vi "Server.vi"() -> ()   [LabVIEW 2023]
uses:
  <vilib>/Utility/file.llb/Read Delimited Spreadsheet (string).vi
  <vilib>/Utility/file.llb/Write Delimited Spreadsheet (string).vi
panel:
  in  "Tab Control":enum32{"CarWash", "Admin"}(tab)
  out "Vehicle Out of Position":bool
  out "Air Dry":bool
  out "Clean Water Rinse":bool
  out "Main High Pressure Wash":bool
  out "Soap Application":bool
  out "Under Body Wash":bool
  in  "Deluxe Wash":bool
  in  "Econony Wash":bool
  in  "Under body\nWash Position\nSwitch":bool
  in  "Main Wash\nPosition\nSwitch":bool
  in  "Air Dry\nPosition\nSwitch":bool
  in  "stop":bool
  out "Timer":i32
  in  "Users":string[][](array[string])
  in  "Read":bool
  in  "Save":bool
  in  "stop 2":bool
  out "Log":bool
  out "Count":bool
  # "Purchase Selection"
  # "Car Wash Indicators"
  # "Car Wash Simulation Switches"
  # "Username"
  # "Password"
  # "Role"
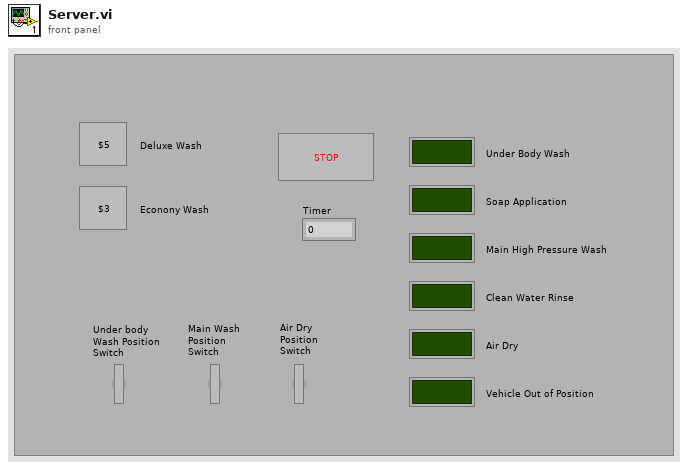
[diagram p1: front panel]
types:
  T1 = enum8{"Enabled", "Disabled", "Disabled and Grayed Out"}
  T2 = enum16{"Innit", "UBW", "SA", "MHPW", "CWR", "ADC"}
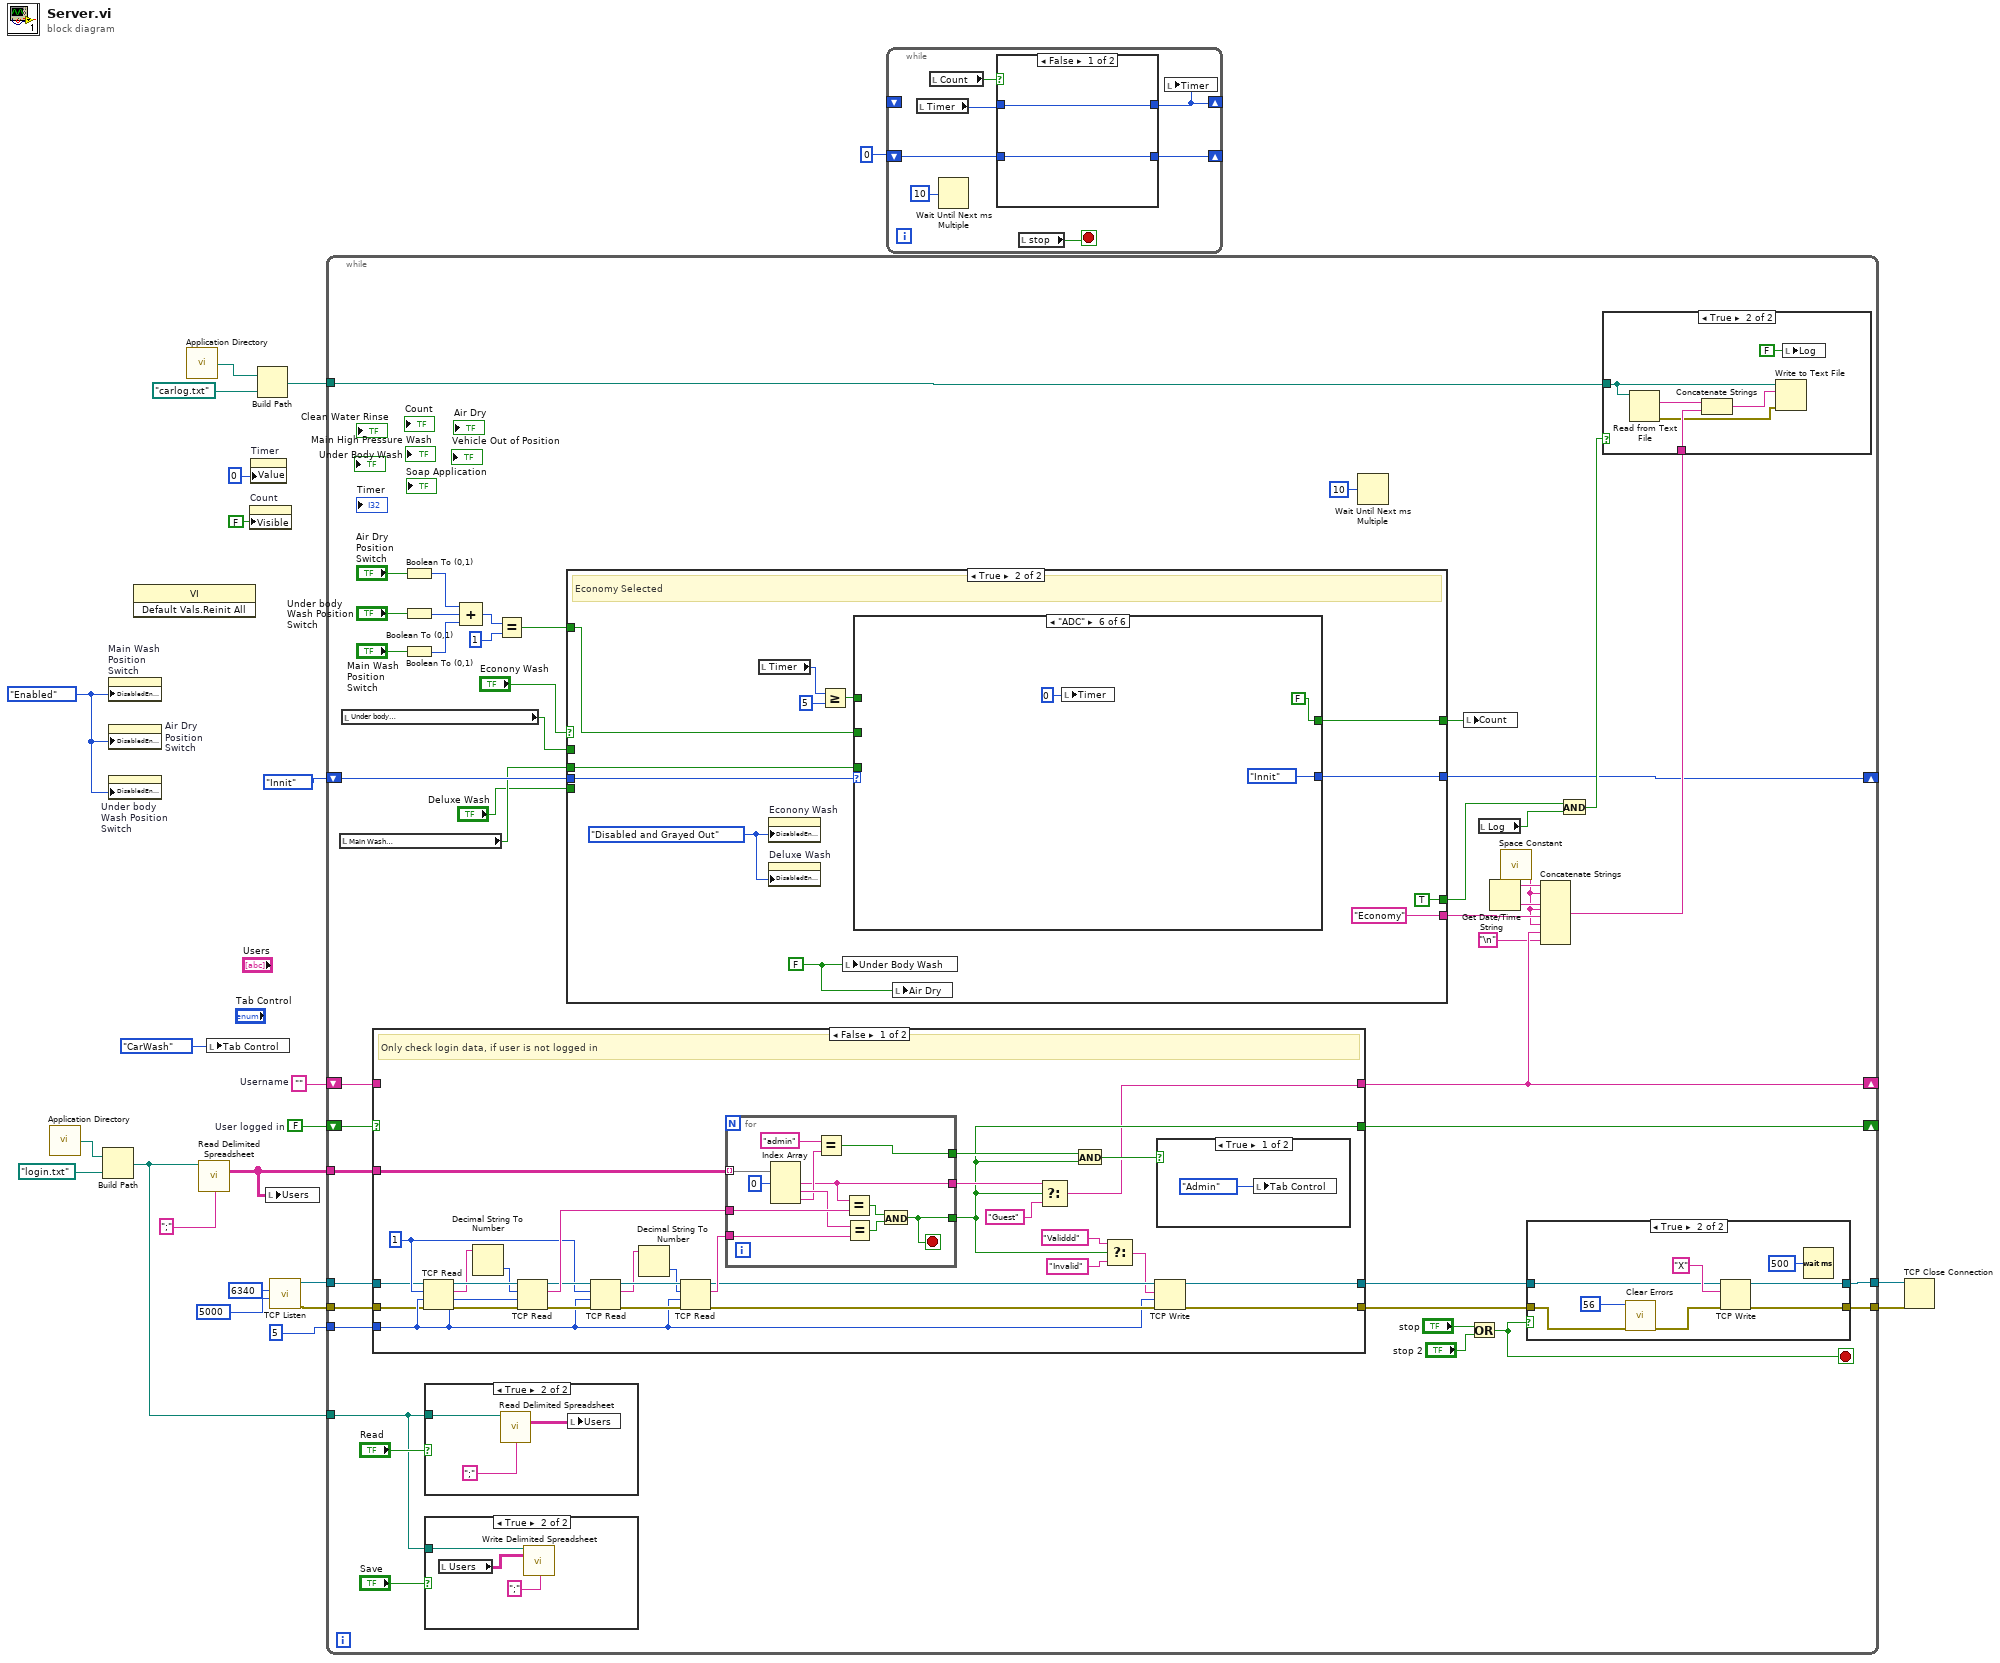
[diagram p0: block diagram]
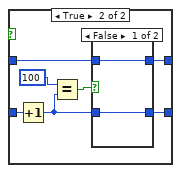
[diagram p2: hidden frame]
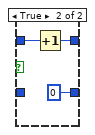
[diagram p3: hidden frame]
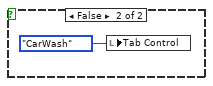
[diagram p6: hidden frame]
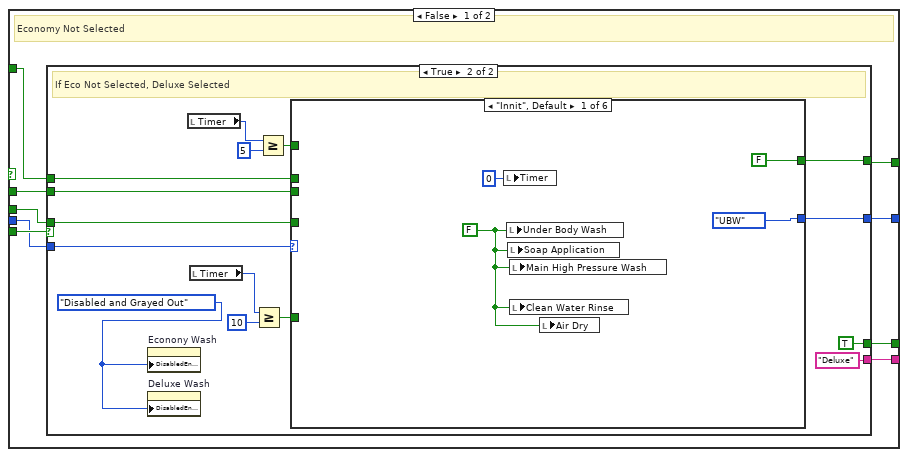
[diagram p10: hidden frame]
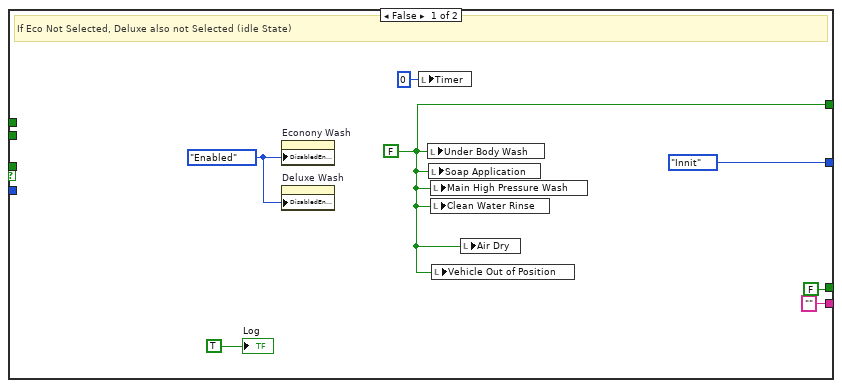
[diagram p11: hidden frame]
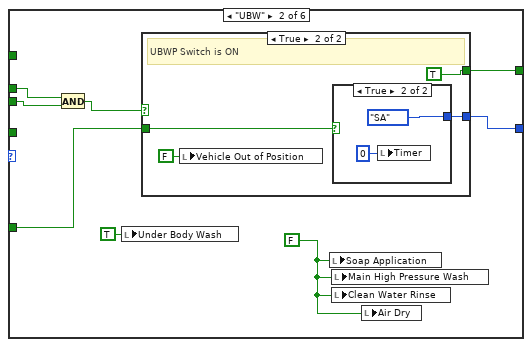
[diagram p12: hidden frame]
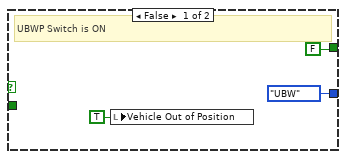
[diagram p13: hidden frame]
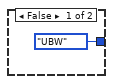
[diagram p14: hidden frame]
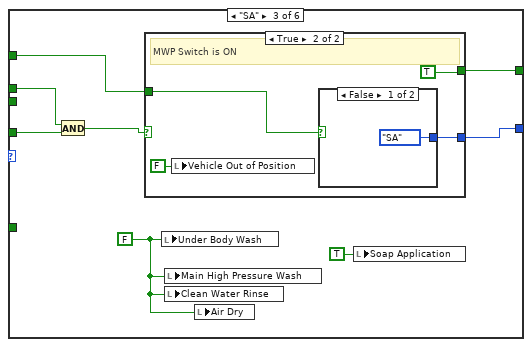
[diagram p15: hidden frame]
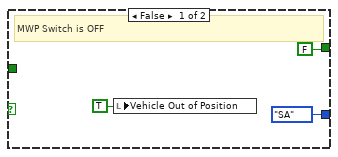
[diagram p16: hidden frame]
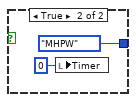
[diagram p17: hidden frame]
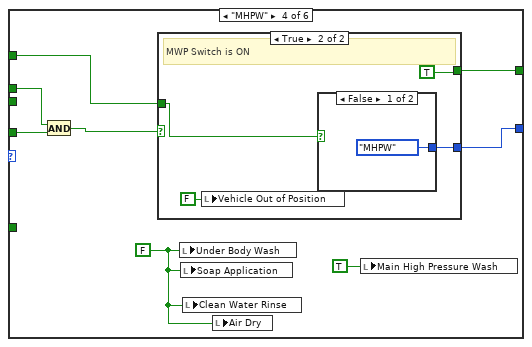
[diagram p18: hidden frame]
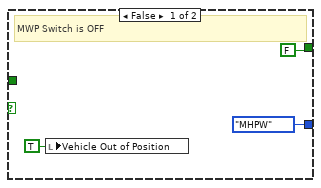
[diagram p19: hidden frame]
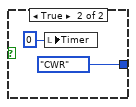
[diagram p20: hidden frame]
diagram:
  w1 = T1."Enabled" ("Disabled")
  w3 = ""  # Username
  w8 = FALSE  # User logged in
  n1 = call <vilib>:"Application Directory.vi"() -> ("Application Directory"=w9:path)
  n2 = Build Path(base path=w9, name or relative path=path "login.txt") -> (appended path=w5:path)
  n3 = property on="Main Wash\nPosition\nSwitch" class="Bool (strict)"("DisabledEnum"=w1) -> ()  [unwired: 2 in, 2 out]
  n4 = property on="Air Dry\nPosition\nSwitch" class="Bool (strict)"("DisabledEnum"=w1) -> ()  [unwired: 2 in, 2 out]
  n5 = property on="Under body\nWash Position\nSwitch" class="Bool (strict)"("DisabledEnum"=w1) -> ()  [unwired: 2 in, 2 out]
  n6 = invoke class="VI" method="Default Vals.Reinit All"() -> ()  [unwired: 3 in, 3 out]
  n7 = call <vilib>:"Application Directory.vi"() -> ("Application Directory"=w13:path)
  n8 = call-poly <vilib>:"Read Delimited Spreadsheet.vi"("file path (dialog if empty)"=w5, "delimiter (\\t)"=";" ("delimiter (\\t)")) -> ("all rows"=w6:string[][])  [unwired: 8 in, 5 out]
  n9 = local write "Tab Control"(enum32{"CarWash", "Admin"}."CarWash" ("Tab Control")) -> ()
  n10 = property on="Count" class="Bool (strict)"("Visible"=FALSE ("Count")) -> ()  [unwired: 2 in, 2 out]
  n11 = property on="Timer" class="DigNum (strict)"("Value"=0 ("Timer")) -> ()  [unwired: 2 in, 2 out]
  n12 = Build Path(base path=w13, name or relative path=path "carlog.txt") -> (appended path=w2:path)
  n13 = local write "Users"(w6) -> ()
  n14 = call <vilib>:"TCP Listen.vi"("timeout ms (wait forever: -1)"=5000 ("timeout ms (60000)"), "port"=u16 6340) -> ("error out"=w16:errorcluster, "connection ID"=w19:refnum<k5>)  [unwired: 5 in, 3 out]
  n15 = while {
    shift-right: [w53] -> _
    shift-left: T2."Innit" -> [w68]
    tunnel: w2 -> [w56]
    tunnel: w19 -> [w51]
    tunnel: [w47] -> w18
    tunnel: [w46] -> w17
    tunnel: w16 -> [w50]
    tunnel: 5 ("timeout ms (60000)") -> [w52]
    shift-right: [w44] -> _
    shift-left: w8 -> [w45]
    tunnel: w6 -> [w43]
    tunnel: w5 -> [w37]
    shift-right: [w34] -> _
    shift-left: w3 -> [w36]
    stop <- w40 stop-if-true
    n16 = local read "Main Wash\nPosition\nSwitch"() -> (w67:bool)
    n17 = local read "Under body\nWash Position\nSwitch"() -> (w66:bool)
    n18 = case shown="False" w45 {
      selector: w45 -> [_ w120]
      tunnel: w52 -> [w86 _]
      tunnel: w51 -> [w85 w122]
      tunnel: w50 -> [w84 w121]
      tunnel: [w83 w121] -> w49
      tunnel: [w82 w122] -> w48
      tunnel: [w77 w120] -> w44
      tunnel: w43 -> [w81 _]
      tunnel: w36 -> [_ w119]
      tunnel: [w75 w119] -> w34
      frame False {
        w87 = 1
        # "Only check login data, if user is not logged in"
        n19 = TCP Read(connection ID=w85, bytes to read=w87, error in (no error)=w84, 9:w86) -> (connection ID out=w97:refnum<k5>, data out=w95:string, error out=w96:errorcluster)  [unwired: 1 in]
        n20 = Decimal String To Number(string=w95) -> (number=w94:i32)  [unwired: 2 in, 1 out]
        n21 = TCP Read(connection ID=w97, bytes to read=w94, error in (no error)=w96, 9:w86) -> (connection ID out=w90:refnum<k5>, data out=w104:string, error out=w91:errorcluster)  [unwired: 1 in]
        n22 = TCP Read(connection ID=w90, bytes to read=w87, error in (no error)=w91, 9:w86) -> (connection ID out=w93:refnum<k5>, data out=w89:string, error out=w92:errorcluster)  [unwired: 1 in]
        n23 = Decimal String To Number(string=w89) -> (number=w88:i32)  [unwired: 2 in, 1 out]
        n24 = TCP Read(connection ID=w93, bytes to read=w88, error in (no error)=w92, 9:w86) -> (connection ID out=w100:refnum<k5>, data out=w103:string, error out=w99:errorcluster)  [unwired: 1 in]
        n25 = for {
          tunnel: w104 -> [w117]
          tunnel: w103 -> [w116]
          tunnel: w81 -> [w118] mode=indexing
          tunnel: [w111] -> w77
          tunnel: [w108] -> w80
          tunnel: [w107] -> w78
          stop <- w111 stop-if-true
          n26 = Index Array(array=w118, index #1=0 ("index")) -> (element #1=w107:string, element #2=w114:string, element #3=w110:string)  [unwired: 2 in]
          n27 = Equal?(x="admin", y=w110) -> (x = y?=w108:bool)
          n28 = Equal?(x=w107, y=w117) -> (x = y?=w112:bool)
          n29 = Equal?(x=w114, y=w116) -> (x = y?=w113:bool)
          n30 = And(x=w112, y=w113) -> (x .and. y?=w111:bool)
        }
        n31 = Select(t=w78, s=w77, f="Guest") -> (s? t:f=w75:string)
        n32 = And(x=w80, y=w77) -> (x .and. y?=w79:bool)
        n33 = Select(t="Validdd", s=w77, f="Invalid") -> (s? t:f=w98:string)
        n34 = TCP Write(connection ID=w100, data in=w98, error in (no error)=w99, 9:w86) -> (connection ID out=w82:refnum<k5>, error out=w83:errorcluster)  [unwired: 1 out]
        n35 = case shown="True" w79 {
          frame True {
            n36 = local write "Tab Control"(enum32{"CarWash", "Admin"}."Admin" ("Tab Control")) -> ()
          }
          frame False {
            n37 = local write "Tab Control"(enum32{"CarWash", "Admin"}."CarWash" ("Tab Control")) -> ()
          }
        }
      }
      frame True {
        # "When logged in, there is nothig to do here"
      }
    }
    n38 = Boolean To (0,1)(Boolean="Air Dry\nPosition\nSwitch") -> (0, 1=w29:i16)
    n39 = Boolean To (0,1)(Boolean="Under body\nWash Position\nSwitch") -> (0, 1=w28:i16)
    n40 = Boolean To (0,1)(Boolean="Main Wash\nPosition\nSwitch") -> (0, 1=w27:i16)
    n41 = case shown="True" "Read" {
      tunnel: w37 -> [_ w72]
      frame False {
      }
      frame True {
        n42 = call-poly <vilib>:"Read Delimited Spreadsheet.vi"("file path (dialog if empty)"=w72, "delimiter (\\t)"=";" ("delimiter (\\t)")) -> ("all rows"=w74:string[][])  [unwired: 8 in, 5 out]
        n43 = local write "Users"(w74) -> ()
      }
    }
    n44 = case shown="True" "Save" {
      tunnel: w37 -> [_ w70]
      frame False {
      }
      frame True {
        n45 = local read "Users"() -> (w69:string[][])
        n46 = call-poly <vilib>:"Write Delimited Spreadsheet.vi"("file path (dialog if empty)"=w70, "2D data"=w69, "delimiter (\\t)"=";" ("delimiter (\\t)")) -> ()  [unwired: 11 in, 2 out]
      }
    }
    n47 = Compound Arithmetic op=ADD(w29, w28, w27) -> (w26:i16)
    n48 = Equal?(x=w26, y=i16 1) -> (x = y?=w24:bool)
    n49 = case shown="True" "Econony Wash" {
      tunnel: w68 -> [w146 w275]
      tunnel: "Deluxe Wash" -> [w147 _]
      tunnel: [w145 w274] -> w53
      tunnel: w67 -> [w143 w272]
      tunnel: w66 -> [w144 _]
      tunnel: [w142 w271] -> w63
      tunnel: [w141 "Economy"] -> w55
      tunnel: [w140 TRUE] -> w54
      tunnel: w24 -> [w139 w264]
      frame False {
        # "Economy Not Selected"
        n50 = case shown="True" w147 {
          tunnel: w146 -> [_ w169]
          tunnel: [T2."Innit" w168] -> w145
          tunnel: w144 -> [_ w167]
          tunnel: w143 -> [_ w166]
          tunnel: [w152 w161] -> w142
          tunnel: ["" "Deluxe"] -> w141
          tunnel: [FALSE TRUE] -> w140
          tunnel: w139 -> [_ w155]
          frame False {
            w148 = T1."Enabled" ("Disabled")
            w152 = FALSE ("Soap Application")
            # "If Eco Not Selected, Deluxe also not Selected (idle State)"
            n51 = property on="Econony Wash" class="Bool (strict)"("DisabledEnum"=w148) -> ()  [unwired: 2 in, 2 out]
            n52 = property on="Deluxe Wash" class="Bool (strict)"("DisabledEnum"=w148) -> ()  [unwired: 2 in, 2 out]
            n53 = local write "Timer"(0 ("Timer")) -> ()
            n54 = local write "Under Body Wash"(w152) -> ()
            n55 = local write "Soap Application"(w152) -> ()
            n56 = local write "Main High Pressure Wash"(w152) -> ()
            n57 = local write "Clean Water Rinse"(w152) -> ()
            n58 = local write "Vehicle Out of Position"(w152) -> ()
            n59 = local write "Air Dry"(w152) -> ()
            "Log" <- TRUE
          }
          frame True {
            w156 = T1."Disabled and Grayed Out" ("Disabled")
            # "If Eco Not Selected, Deluxe Selected"
            n60 = property on="Econony Wash" class="Bool (strict)"("DisabledEnum"=w156) -> ()  [unwired: 2 in, 2 out]
            n61 = property on="Deluxe Wash" class="Bool (strict)"("DisabledEnum"=w156) -> ()  [unwired: 2 in, 2 out]
            n62 = local read "Timer"() -> (w163:i32)
            n63 = local read "Timer"() -> (w162:i32)
            n64 = Greater Or Equal?(x=w162, y=10) -> (x >= y?=w160:bool)
            n65 = Greater Or Equal?(x=w163, y=5) -> (x >= y?=w159:bool)
            n66 = case shown="\"Innit\", Default" w169 {
              tunnel: [T2."UBW" w181 w199 w217 w234 w253] -> w168
              tunnel: w167 -> [_ w176 _ _ _ _]
              tunnel: w166 -> [_ _ w194 w212 w230 _]
              tunnel: [FALSE w178 w196 w214 w232 w249] -> w161
              tunnel: w160 -> [_ w177 _ _ _ w250]
              tunnel: w159 -> [_ _ w195 w213 w231 _]
              tunnel: w155 -> [_ w175 w192 w210 w228 w246]
              frame "Innit", Default {
                w172 = FALSE ("Soap Application")
                n67 = local write "Timer"(0 ("Timer")) -> ()
                n68 = local write "Under Body Wash"(w172) -> ()
                n69 = local write "Soap Application"(w172) -> ()
                n70 = local write "Main High Pressure Wash"(w172) -> ()
                n71 = local write "Clean Water Rinse"(w172) -> ()
                n72 = local write "Air Dry"(w172) -> ()
              }
              frame "UBW" {
                w179 = FALSE ("Soap Application")
                n73 = And(x=w175, y=w176) -> (x .and. y?=w174:bool)
                n74 = local write "Under Body Wash"(TRUE ("Soap Application")) -> ()
                n75 = case shown="True" w174 {
                  tunnel: [T2."UBW" w188] -> w181
                  tunnel: [FALSE TRUE] -> w178
                  tunnel: w177 -> [_ w185]
                  frame False {
                    # "UBWP Switch is ON"
                    n76 = local write "Vehicle Out of Position"(TRUE ("Vehicle Out of Position")) -> ()
                  }
                  frame True {
                    # "UBWP Switch is ON"
                    n77 = local write "Vehicle Out of Position"(FALSE ("Vehicle Out of Position")) -> ()
                    n78 = case shown="True" w185 {
                      tunnel: [T2."UBW" T2."SA"] -> w188
                      frame False {
                      }
                      frame True {
                        n79 = local write "Timer"(0 ("Timer")) -> ()
                      }
                    }
                  }
                }
                n80 = local write "Soap Application"(w179) -> ()
                n81 = local write "Main High Pressure Wash"(w179) -> ()
                n82 = local write "Clean Water Rinse"(w179) -> ()
                n83 = local write "Air Dry"(w179) -> ()
              }
              frame "SA" {
                w198 = FALSE ("Soap Application")
                n84 = And(x=w192, y=w194) -> (x .and. y?=w193:bool)
                n85 = case shown="True" w193 {
                  tunnel: [T2."SA" w206] -> w199
                  tunnel: [FALSE TRUE] -> w196
                  tunnel: w195 -> [_ w203]
                  frame False {
                    # "MWP Switch is OFF"
                    n86 = local write "Vehicle Out of Position"(TRUE ("Vehicle Out of Position")) -> ()
                  }
                  frame True {
                    # "MWP Switch is ON"
                    n87 = local write "Vehicle Out of Position"(FALSE ("Vehicle Out of Position")) -> ()
                    n88 = case shown="False" w203 {
                      tunnel: [T2."SA" T2."MHPW"] -> w206
                      frame False {
                      }
                      frame True {
                        n89 = local write "Timer"(0 ("Timer")) -> ()
                      }
                    }
                  }
                }
                n90 = local write "Under Body Wash"(w198) -> ()
                n91 = local write "Main High Pressure Wash"(w198) -> ()
                n92 = local write "Clean Water Rinse"(w198) -> ()
                n93 = local write "Air Dry"(w198) -> ()
                n94 = local write "Soap Application"(TRUE ("Soap Application")) -> ()
              }
              frame "MHPW" {
                w216 = FALSE ("Soap Application")
                n95 = And(x=w210, y=w212) -> (x .and. y?=w211:bool)
                n96 = case shown="True" w211 {
                  tunnel: [T2."MHPW" w224] -> w217
                  tunnel: [FALSE TRUE] -> w214
                  tunnel: w213 -> [_ w221]
                  frame False {
                    # "MWP Switch is OFF"
                    n97 = local write "Vehicle Out of Position"(TRUE ("Vehicle Out of Position")) -> ()
                  }
                  frame True {
                    # "MWP Switch is ON"
                    n98 = local write "Vehicle Out of Position"(FALSE ("Vehicle Out of Position")) -> ()
                    n99 = case shown="False" w221 {
                      tunnel: [T2."MHPW" T2."CWR"] -> w224
                      frame False {
                      }
                      frame True {
                        n100 = local write "Timer"(0) -> ()
                      }
                    }
                  }
                }
                n101 = local write "Under Body Wash"(w216) -> ()
                n102 = local write "Soap Application"(w216) -> ()
                n103 = local write "Clean Water Rinse"(w216) -> ()
                n104 = local write "Air Dry"(w216) -> ()
                n105 = local write "Main High Pressure Wash"(TRUE ("Soap Application")) -> ()
              }
              frame "CWR" {
                w233 = FALSE ("Soap Application")
                n106 = And(x=w228, y=w230) -> (x .and. y?=w229:bool)
                n107 = local write "Clean Water Rinse"(TRUE ("Soap Application")) -> ()
                n108 = local write "Under Body Wash"(w233) -> ()
                n109 = local write "Soap Application"(w233) -> ()
                n110 = local write "Main High Pressure Wash"(w233) -> ()
                n111 = local write "Air Dry"(w233) -> ()
                n112 = case shown="True" w229 {
                  tunnel: [T2."CWR" w242] -> w234
                  tunnel: [FALSE TRUE] -> w232
                  tunnel: w231 -> [_ w239]
                  frame False {
                    # "MWP Switch is OFF"
                    n113 = local write "Vehicle Out of Position"(TRUE ("Vehicle Out of Position")) -> ()
                  }
                  frame True {
                    # "MWP Switch is ON"
                    n114 = local write "Vehicle Out of Position"(FALSE ("Vehicle Out of Position")) -> ()
                    n115 = case shown="True" w239 {
                      tunnel: [T2."CWR" T2."ADC"] -> w242
                      frame False {
                      }
                      frame True {
                        n116 = local write "Timer"(0 ("Timer")) -> ()
                      }
                    }
                  }
                }
              }
              frame "ADC" {
                w252 = FALSE ("Soap Application")
                n117 = local read "Air Dry\nPosition\nSwitch"() -> (w248:bool)
                n118 = local write "Under Body Wash"(w252) -> ()
                n119 = local write "Soap Application"(w252) -> ()
                n120 = local write "Main High Pressure Wash"(w252) -> ()
                n121 = local write "Clean Water Rinse"(w252) -> ()
                n122 = local write "Air Dry"(TRUE ("Soap Application")) -> ()
                n123 = And(x=w246, y=w248) -> (x .and. y?=w247:bool)
                n124 = case shown="True" w247 {
                  tunnel: [T2."ADC" w260] -> w253
                  tunnel: w250 -> [_ w258]
                  tunnel: [FALSE TRUE] -> w249
                  frame False {
                    n125 = local write "Vehicle Out of Position"(TRUE ("Vehicle Out of Position")) -> ()
                  }
                  frame True {
                    n126 = local write "Vehicle Out of Position"(FALSE ("Vehicle Out of Position")) -> ()
                    n127 = case shown="True" w258 {
                      tunnel: [T2."ADC" T2."Innit"] -> w260
                      frame False {
                      }
                      frame True {
                        n128 = invoke class="VI" method="Default Vals.Reinit All"() -> ()  [unwired: 3 in, 3 out]
                        n129 = local write "Timer"(0 ("Timer")) -> ()
                      }
                    }
                  }
                }
              }
            }
          }
        }
      }
      frame True {
        w265 = T1."Disabled and Grayed Out" ("Disabled")
        w273 = FALSE ("Soap Application")
        # "Economy Selected"
        n130 = local read "Timer"() -> (w270:i32)
        n131 = property on="Econony Wash" class="Bool (strict)"("DisabledEnum"=w265) -> ()  [unwired: 2 in, 2 out]
        n132 = property on="Deluxe Wash" class="Bool (strict)"("DisabledEnum"=w265) -> ()  [unwired: 2 in, 2 out]
        n133 = Greater Or Equal?(x=w270, y=5) -> (x >= y?=w268:bool)
        n134 = local write "Under Body Wash"(w273) -> ()
        n135 = case shown="\"ADC\"" w275 {
          tunnel: [T2."SA" T2."Innit" w290 w308 w326 T2."Innit"] -> w274
          tunnel: w272 -> [_ _ w285 w303 w321 _]
          tunnel: [FALSE ("Count") FALSE ("Count") w287 w305 w322 FALSE ("Count")] -> w271
          tunnel: w268 -> [_ _ w286 w304 w323 _]
          tunnel: w264 -> [_ _ w284 w302 w319 _]
          frame "Innit", Default {
            w278 = FALSE ("Soap Application")
            n136 = local write "Main High Pressure Wash"(w278) -> ()
            n137 = local write "Clean Water Rinse"(w278) -> ()
            n138 = local write "Soap Application"(w278) -> ()
            n139 = local write "Timer"(0 ("Timer")) -> ()
          }
          frame "UBW" {
            n140 = local write "Timer"(0 ("Timer")) -> ()
          }
          frame "SA" {
            w288 = FALSE ("Soap Application")
            n141 = And(x=w284, y=w285) -> (x .and. y?=w283:bool)
            n142 = local write "Soap Application"(TRUE ("Soap Application")) -> ()
            n143 = local write "Main High Pressure Wash"(w288) -> ()
            n144 = case shown="True" w283 {
              tunnel: [T2."SA" w297] -> w290
              tunnel: [FALSE ("Count") TRUE ("Count")] -> w287
              tunnel: w286 -> [_ w294]
              frame False {
                # "MWP Switch is OFF"
                n145 = local write "Vehicle Out of Position"(TRUE ("Vehicle Out of Position")) -> ()
              }
              frame True {
                # "MWP Switch is ON"
                n146 = local write "Vehicle Out of Position"(FALSE ("Vehicle Out of Position")) -> ()
                n147 = case shown="False" w294 {
                  tunnel: [T2."SA" T2."MHPW"] -> w297
                  frame False {
                  }
                  frame True {
                    n148 = local write "Timer"(0 ("Timer")) -> ()
                  }
                }
              }
            }
            n149 = local write "Clean Water Rinse"(w288) -> ()
          }
          frame "MHPW" {
            w307 = FALSE ("Soap Application")
            n150 = local write "Main High Pressure Wash"(TRUE ("Soap Application")) -> ()
            n151 = And(x=w302, y=w303) -> (x .and. y?=w301:bool)
            n152 = local write "Clean Water Rinse"(w307) -> ()
            n153 = local write "Soap Application"(w307) -> ()
            n154 = case shown="False" w301 {
              tunnel: [T2."MHPW" w315] -> w308
              tunnel: [FALSE TRUE] -> w305
              tunnel: w304 -> [_ w312]
              frame False {
                # "MWP Switch is OFF"
                n155 = local write "Vehicle Out of Position"(TRUE ("Vehicle Out of Position")) -> ()
              }
              frame True {
                # "MWP Switch is ON"
                n156 = local write "Vehicle Out of Position"(FALSE ("Vehicle Out of Position")) -> ()
                n157 = case shown="True" w312 {
                  tunnel: [T2."MHPW" T2."CWR"] -> w315
                  frame False {
                  }
                  frame True {
                    n158 = local write "Timer"(0 ("Timer")) -> ()
                  }
                }
              }
            }
          }
          frame "CWR" {
            w324 = FALSE ("Soap Application")
            n159 = local write "Clean Water Rinse"(TRUE ("Soap Application")) -> ()
            n160 = And(x=w319, y=w321) -> (x .and. y?=w320:bool)
            n161 = local write "Main High Pressure Wash"(w324) -> ()
            n162 = local write "Soap Application"(w324) -> ()
            n163 = case shown="True" w320 {
              tunnel: [T2."CWR" w333] -> w326
              tunnel: w323 -> [_ w331]
              tunnel: [FALSE TRUE] -> w322
              frame False {
                # "MWP Switch is OFF"
                n164 = local write "Vehicle Out of Position"(TRUE ("Vehicle Out of Position")) -> ()
              }
              frame True {
                # "MWP Switch is ON"
                n165 = local write "Vehicle Out of Position"(FALSE ("Vehicle Out of Position")) -> ()
                n166 = case shown="True" w331 {
                  tunnel: [T2."CWR" T2."Innit"] -> w333
                  frame False {
                  }
                  frame True {
                    n167 = invoke class="VI" method="Default Vals.Reinit All"() -> ()  [unwired: 3 in, 3 out]
                    n168 = local write "Timer"(0 ("Timer")) -> ()
                  }
                }
              }
            }
          }
          frame "ADC" {
            n169 = local write "Timer"(0 ("Timer")) -> ()
          }
        }
        n170 = local write "Air Dry"(w273) -> ()
      }
    }
    n171 = Wait Until Next ms Multiple(millisecond multiple=u32 10) -> ()  [unwired: 1 out]
    n172 = local write "Count"(w63) -> ()
    n173 = Or(x="stop", y="stop 2") -> (x .or. y?=w40:bool)
    n174 = local read "Log"() -> (w60:bool)
    n175 = Get Date/Time String() -> (date string=w59:string, time string=w58:string)  [unwired: 3 in]
    n176 = call <vilib>:"Space Constant.vi"() -> ("String"=w35:string)
    n177 = case shown="True" w40 {
      tunnel: w49 -> [w123 w132]
      tunnel: w48 -> [w124 w126]
      tunnel: [w124 w131] -> w47
      tunnel: [w123 w130] -> w46
      frame False {
      }
      frame True {
        n178 = call <vilib>:"Clear Errors.vi"("error in (no error)"=w132, "specific error code to clear (0: all)"=56) -> ("error out"=w127:errorcluster)  [unwired: 4 in, 1 out]
        n179 = TCP Write(connection ID=w126, data in="X", error in (no error)=w127) -> (connection ID out=w131:refnum<k5>, error out=w130:errorcluster)  [unwired: 1 in, 1 out]
        n180 = Wait (ms)(milliseconds to wait=u32 500) -> ()  [unwired: 1 out]
      }
    }
    n181 = Concatenate Strings(w59, w35, w58, w35, w55, w35, w34, "\n") -> (w57:string)
    n182 = And(x=w54, y=w60) -> (x .and. y?=w61:bool)
    n183 = case shown="True" w61 {
      tunnel: w57 -> [_ w137]
      tunnel: w56 -> [_ w135]
      frame False {
      }
      frame True {
        n184 = Read from Text File(file (use dialog)=w135) -> (text=w133:string, error out=w134:errorcluster)  [unwired: 3 in, 2 out]
        n185 = Concatenate Strings "Concatenate Strings"(w133, w137) -> (w136:string)
        n186 = Write to Text File(file (use dialog)=w135, text=w136, error in=w134) -> ()  [unwired: 1 in, 3 out]
        n187 = local write "Log"(FALSE ("Log")) -> ()
      }
    }
  }
  n188 = while {
    shift-right: [w346] -> _
    shift-left: 0 -> [w343]
    shift-right: [w341] -> _
    shift-left: _ -> [_]
    stop <- w345 stop-if-true
    n189 = local read "Timer"() -> (w340:i32)
    n190 = local read "Count"() -> (w344:bool)
    n191 = Wait Until Next ms Multiple(millisecond multiple=u32 10) -> ()  [unwired: 1 out]
    n192 = case shown="False" w344 {
      tunnel: w343 -> [w347 w355]
      tunnel: [w347 w351] -> w346
      tunnel: w340 -> [w348 w350]
      tunnel: [w348 w349] -> w341
      frame False {
      }
      frame True {
        n193 = Increment(x=w355) -> (x+1=w352:i32)
        n194 = Equal?(x=100, y=w352) -> (x = y?=w353:bool)
        n195 = case shown="False" w353 {
          tunnel: w352 -> [w357 _]
          tunnel: [w357 0] -> w351
          tunnel: w350 -> [w356 w358]
          tunnel: [w356 w359] -> w349
          frame False {
          }
          frame True {
            n196 = Increment(x=w358) -> (x+1=w359:i32)
          }
        }
      }
    }
    n197 = local read "stop"() -> (w345:bool)
    n198 = local write "Timer"(w341) -> ()
  }
  n199 = TCP Close Connection(connection ID=w18, error in (no error)=w17) -> ()  [unwired: 1 in, 2 out]
